vi "Ex2Task3.vi"() -> ()   [LabVIEW 2014, in "Diaz_Razo_5th_LegoRobotics_11-29-16.lvrbt"]
uses:
  Diaz_Razo_5th_LegoRobotics_11-29-16.lvrbt
panel:
  out "Average Value":dbl
  out "Waveform Graph":dbl[](graph)
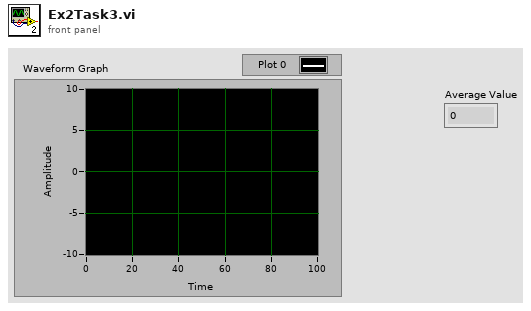
[diagram p1: front panel]
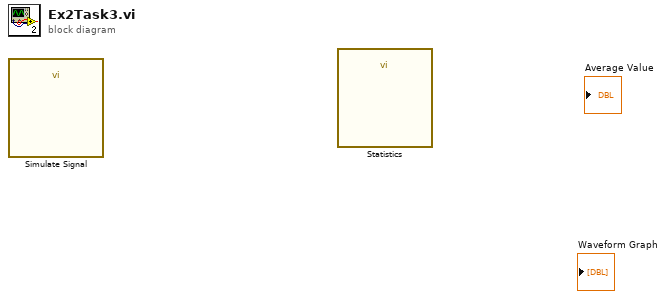
[diagram p0: block diagram]
diagram:
  n1 = call "Simulate Signal"() -> ()  [unwired: 14 in, 2 out]
  n2 = call "Statistics"() -> ()  [unwired: 26 in, 2 out]
